vi "Main.vi"(8 "error in (no error)":errorcluster) -> ()   [LabVIEW 2018, in "Main.lvlib"]
uses:
  Main.lvlib
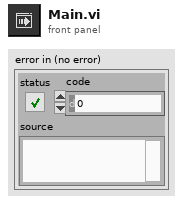
[diagram p1: front panel]
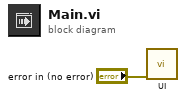
[diagram p0: block diagram]
diagram:
  n1 = call "UI.vi"("error in (no error)"="error in (no error)") -> ()  [unwired: 10 in, 1 out]
